vi "Process Modbus Coils.vi"(8 "error in":errorcluster, 11 "Alabama Power Remote":refnum<class "Alabama Power Remote.lvclass">) -> (0 "error out":errorcluster, 3 "dup Alabama Power Remote":refnum<class "Alabama Power Remote.lvclass">)   [LabVIEW 2018, in "Alabama Power Remote Actor.lvlib" / "Alabama Power Remote.lvclass"]
uses:
  Alabama Power Remote.lvclass
  C:/Users/Administrator/Desktop/2018LabVIEW EMS/Remote Operation/Remote Operation Abstract/Remote Operation Abstract.lvclass
  Alabama Power Remote.lvclass/Alabama Power Remote.ctl
  <vilib>/ActorFramework/Actor/Actor.lvclass/Actor.ctl
  Remote Operation Abstract/Remote Operation Abstract.lvclass/Remote Operation Abstract.ctl
  Remote Operation Abstract Messages/Resynchronize Microgrid Msg/Resynchronize Microgrid Msg.lvclass/Resynchronize Microgrid Msg.ctl
  <vilib>/ActorFramework/Message Enqueuer/Message Enqueuer.lvclass/Message Enqueuer.ctl
  Remote Operation Abstract Messages/Island Microgrid Msg/Island Microgrid Msg.lvclass/Island Microgrid Msg.ctl
  <vilib>/ActorFramework/Actor/Read Caller Enqueuer.vi
  Remote Operation Abstract Messages/Resynchronize Microgrid Msg/Send Resynchronize Microgrid.vi
  Remote Operation Abstract Messages/Island Microgrid Msg/Send Island Microgrid.vi
  <vilib>/ActorFramework/Message Enqueuer/Enqueue.vi
  Remote Operation Abstract/Remote Operation Abstract.lvclass
  C:/Program Files (x86)/National Instruments/LabVIEW 2018/vi.lib/ActorFramework/Actor/Actor.lvclass
  Remote Operation Abstract Messages/Resynchronize Microgrid Msg/Resynchronize Microgrid Msg.lvclass
  C:/Program Files (x86)/National Instruments/LabVIEW 2018/vi.lib/ActorFramework/Message/Message.lvclass
  Remote Operation Abstract Messages/Island Microgrid Msg/Island Microgrid Msg.lvclass
  <vilib>/ActorFramework/Message Priority Queue/Priority Enqueue.vi
  <vilib>/Modbus/master/Modbus Master.lvclass
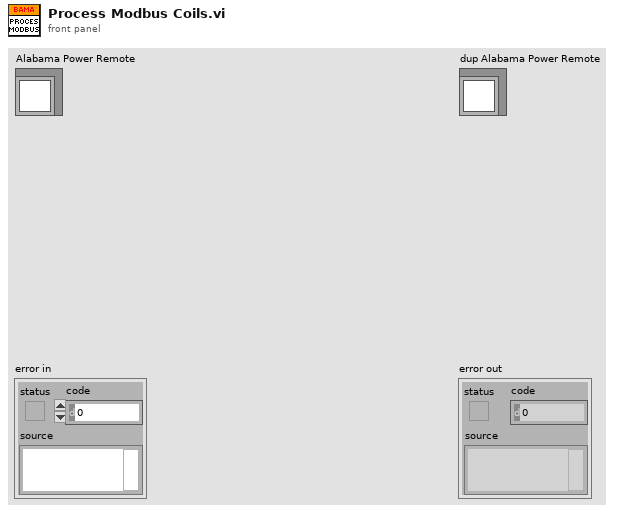
[diagram p1: front panel]
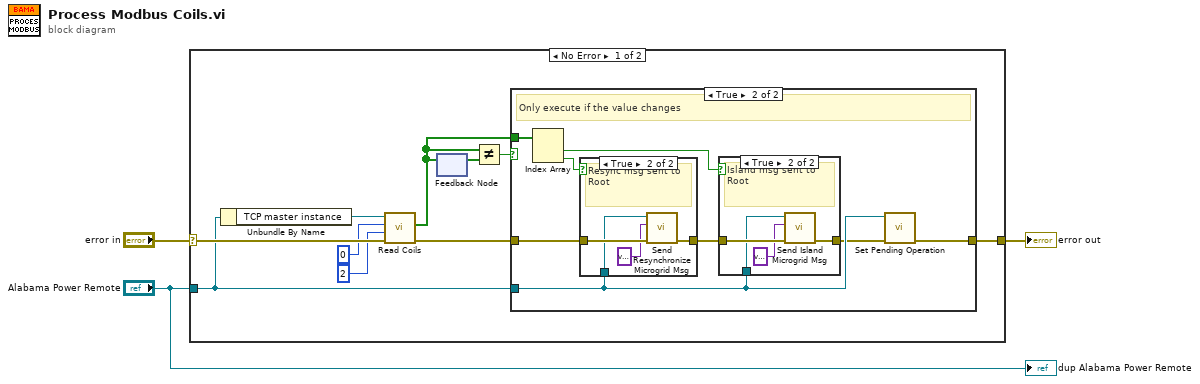
[diagram p0: block diagram]
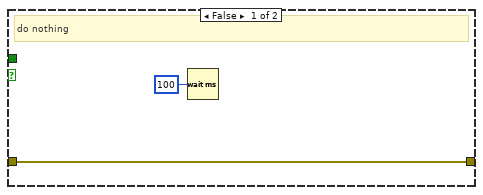
[diagram p2: hidden frame]
diagram:
  n1 = case shown="No Error" "error in" {
    selector: "error in" -> [w12 w34]
    tunnel: [w4 w34] -> w2
    tunnel: "Alabama Power Remote" -> [w5 _]
    frame No Error {
      n2 = Unbundle By Name(w5) -> ("TCP master instance"=w13:refnum<class "Modbus Master.lvclass">)
      n3 = call-dynamic "Read Coils.vi"("error in (no error)"=w12, "number of coils"=u16 2 ("number of holding registers"), "starting address"=u16 0 ("address"), "Modbus master in"=w13) -> ("error out"=w6:errorcluster, "coil values"=w7:bool[])  [unwired: 5 in, 1 out]
      n4 = feedback #1() -> (w9:bool[])  [unwired: 1 in]
      n5 = feedback-in #1(w7) -> ()
      n6 = Not Equal?(x=w7, y=w9) -> (x != y?=w8:bool)
      n7 = case shown="True" w8 {
        tunnel: w7 -> [_ w22]
        tunnel: w6 -> [w15 w23]
        tunnel: w5 -> [_ w18]
        tunnel: [w15 w16] -> w4
        frame False {
          # "do nothing"
          n8 = Wait (ms)(milliseconds to wait=u32 100) -> ()  [unwired: 1 out]
        }
        frame True {
          # "Only execute if the value changes"
          n9 = Index Array(array=w22) -> (element #1=w19:bool, element #2=w20:bool)  [unwired: 2 in]
          n10 = case shown="True" w20 {
            tunnel: w23 -> [w29 w32]
            tunnel: [w29 w33] -> w21
            tunnel: w18 -> [_ w31]
            frame False {
              # "Do nothing"
            }
            frame True {
              # "Resync msg sent to Root"
              n11 = call "Send Resynchronize Microgrid Msg.vi"("error in"=w32, "Data"=variant, "Remote Operation Abstract in"=w31) -> ("error out"=w33:errorcluster)  [unwired: 7 in, 1 out]
            }
          }
          n12 = case shown="True" w19 {
            tunnel: w21 -> [w24 w28]
            tunnel: w18 -> [_ w27]
            tunnel: [w24 w26] -> w17
            frame False {
              # "Do nothing"
            }
            frame True {
              # "Island msg sent to Root"
              n13 = call "Send Island Microgrid Msg.vi"("error in"=w28, "Data"=variant, "Remote Operation Abstract"=w27) -> ("error out"=w26:errorcluster)  [unwired: 7 in, 1 out]
            }
          }
          n14 = call "Set Pending Operation.vi"("error in"=w17, "Remote Operation Abstract"=w18) -> ("error out"=w16:errorcluster)  [unwired: 8 in, 1 out]
        }
      }
    }
    frame Error {
    }
  }
  "error out" <- w2
  "dup Alabama Power Remote" <- "Alabama Power Remote"
